vi "BodeMagnitudePlot.vi"() -> ()   [LabVIEW 2014]
uses:
  <vilib>/Analysis/NI_AALPro.lvlib
panel:
  out "output cluster":cluster{dbl, dbl}={485.0, -4.636400317630035}
  out "Bode Magnitude Plot":cluster{dbl, dbl}[](graph)=[{10.0, -0.005012263234203178}, {35.0, -0.004334288088328031}, {60.0, -0.052469183684286505}, {85.0, -0.14708259513454006}, {110.0, -0.2852994731890425}, {135.0, -0.4635691718487487}, {160.0, -0.6762171944346845}, {185.0, -0.9184401622526503}, {210.0, -1.1850910297028452}, {235.0, -1.4706596920725958}, {260.0, -1.7709475205952834}, {285.0, -2.08209195433784}, {310.0, -2.4001690568474783}, {335.0, -2.7219697461118812}, {360.0, -3.0461616305738333}, {385.0, -3.369717809528669}, {410.0, -3.691834970075307}, {435.0, -4.010777915884752}, {460.0, -4.325669997460676}, {485.0, -4.636400317630035}]
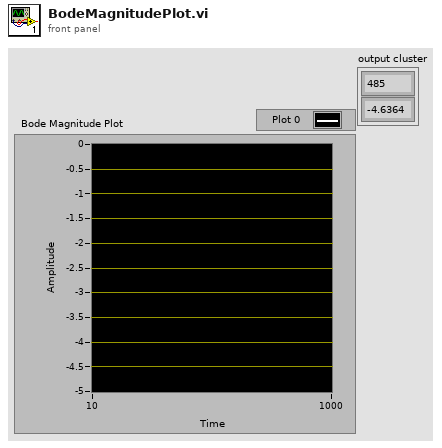
[diagram p1: front panel]
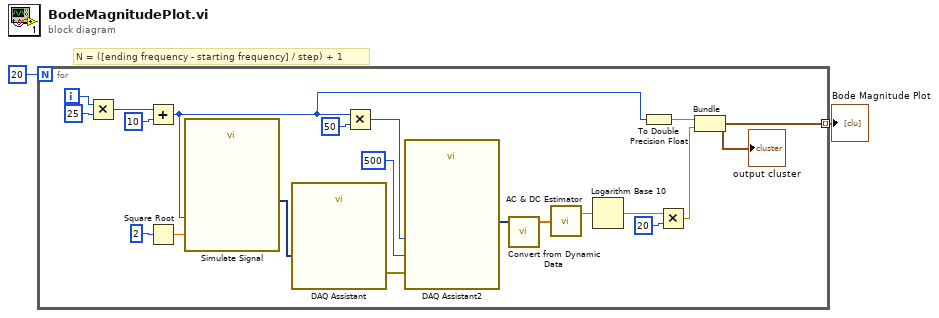
[diagram p0: block diagram]
diagram:
  # "N = ([ending frequency - starting frequency] / step) + 1"
  n1 = for {
    N: 20 -> [_]
    tunnel: [w4] -> w1 mode=indexing
    i -> [w8]
    n2 = Multiply(x=w8, y=25) -> (x*y=w14:i32)
    n3 = Add(x=w14, y=10) -> (x+y=w3:i32)
    n4 = Square Root(x=2) -> (sqrt(x)=w17:dbl)
    n5 = call "Simulate Signal"("Frequency"=w3, "Amplitude"=w17) -> ("Sine"=w10:dynamicdata)  [unwired: 12 in, 1 out]
    n6 = call "DAQ Assistant"("data"=w10) -> ("error out"=w19:errorcluster)  [unwired: 16 in, 2 out]
    n7 = Multiply(x=w3, y=50) -> (x*y=w6:i32)
    n8 = call "DAQ Assistant2"("rate"=w6, "number of samples"=500, "error in"=w19) -> ("data"=w21:dynamicdata)  [unwired: 14 in, 2 out]
    n9 = call "Convert from Dynamic Data"("Dynamic Data Type"=w21) -> ("Array"=w22:dbl[])  [unwired: 3 in]
    n10 = call <vilib>:"AC & DC Estimator.vi"("Signal (V)"=w22) -> ("AC estimate (Vrms)"=w9:dbl)  [unwired: 1 out]
    n11 = Logarithm Base 10(1:w9) -> (0:w11:dbl)
    n12 = To Double Precision Float(number=w3) -> (double precision float=w5:dbl)
    n13 = Multiply(x=w11, y=20) -> (x*y=w7:dbl)
    n14 = Bundle(w5, w7) -> (w4:cluster{dbl, dbl})  [unwired: 1 in]
    "output cluster" <- w4
  }
  "Bode Magnitude Plot" <- w1
